vi "FLDA.vi"(10 "NonTarget":dbl[][](array[numeric]), 11 "Target":dbl[][](array[numeric])) -> (3 "A * B 2":T1)   [LabVIEW 2013]
uses:
  <vilib>/Analysis/Matrix/Datatypes/RealMatrix.ctl
  <vilib>/Analysis/Matrix/NI_Matrix.lvlib
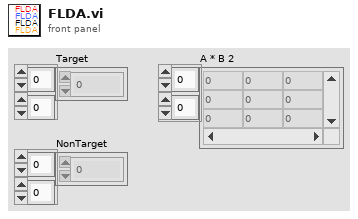
[diagram p1: front panel]
types:
  T1 = typedef "NI_Matrix.lvlib/RealMatrix.ctl" = dbl[][]
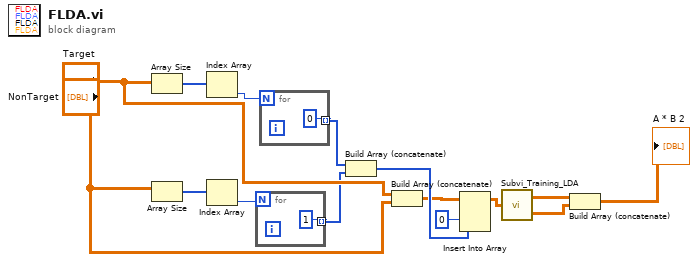
[diagram p0: block diagram]
diagram:
  n1 = Array Size(array="Target") -> (size(s)=w6:i32[])
  n2 = Array Size(array="NonTarget") -> (size(s)=w5:i32[])
  n3 = Index Array(array=w6) -> (element=w4:i32)  [unwired: 1 in]
  n4 = Index Array(array=w5) -> (element=w3:i32)  [unwired: 1 in]
  n5 = for {
    N: w3 -> [_]
    tunnel: [1] -> w1 mode=indexing
  }
  n6 = for {
    N: w4 -> [_]
    tunnel: [0] -> w2 mode=indexing
  }
  n7 = Build Array (concatenate)(w2, w1) -> (w9:i32[])
  n8 = Build Array (concatenate)("Target", "NonTarget") -> (w8:dbl[][])
  n9 = Insert Into Array(array=w8, index (col)=0 ("비활성화된 인덱스 (열)"), new element=w9) -> (w10:dbl[][])  [unwired: 1 in]
  n10 = call "Subvi_Training_LDA.vi"("Input_Data"=w10) -> ("A * B 2"=w12:T1, "A * B"=w11:T1)
  n11 = Build Array (concatenate)(w11, w12) -> (→"A * B 2":T1)
